vi "RT Loop - System Health and FPGA Monitoring.vi"(10 "FPGA VI Reference":T1, 11 "Message Queue":refnum<queue>) -> ()   [LabVIEW 2018]
uses:
  controls/FPGA VI Reference.ctl
  support/Message Queue/Message Cluster (string).ctl
  controls/FPGA State.ctl
  controls/Raw Values.ctl
  Globals/Global - Configuration Options.vi
  Globals/Global - All RT Loop Stop.vi
  <vilib>/Utility/error.llb/Error Cluster From Error Code.vi
  <vilib>/rvi/errors/niLvFpgaAdjustHostInterfaceError.vi
  <vilib>/nisyscfg/Close (System).vi
  <vilib>/rvi/interface/nirviReadWriteControl/nirviReadWriteControl.xnode
  <vilib>/NI_Real-Time Target Support.lvlib
  <vilib>/nisyscfg/nisyscfg.lvlib
  <resource>/objmgr/nisysapi.rc
  NiFpgaLv.dll
  <vilib>/rvi/interface/Simulation/niFpgaSimulationCallBeginRW.vi
  support/Message Queue/Message Queue.lvlib
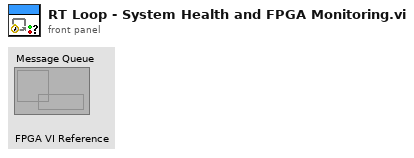
[diagram p1: front panel]
types:
  T1 = typedef "FPGA VI Reference.ctl" = refnum<k20>
  T2 = cluster{"Channel 0":fxp<+/-,20,5>, "Channel 1":fxp<+/-,20,5>, "Channel 2":bool}
  T3 = typedef "NI_Real-Time Target Support.lvlib/RT CPU Load.ctl" = cluster{"Total (%)":dbl, "Time Critical (%)":dbl, "Timed Structures (%)":dbl, "High (%)":dbl, "Above Normal (%)":dbl, "Normal (%)":dbl, "Background (%)":dbl, "Idle (%)":dbl, "ISR (%)":dbl}
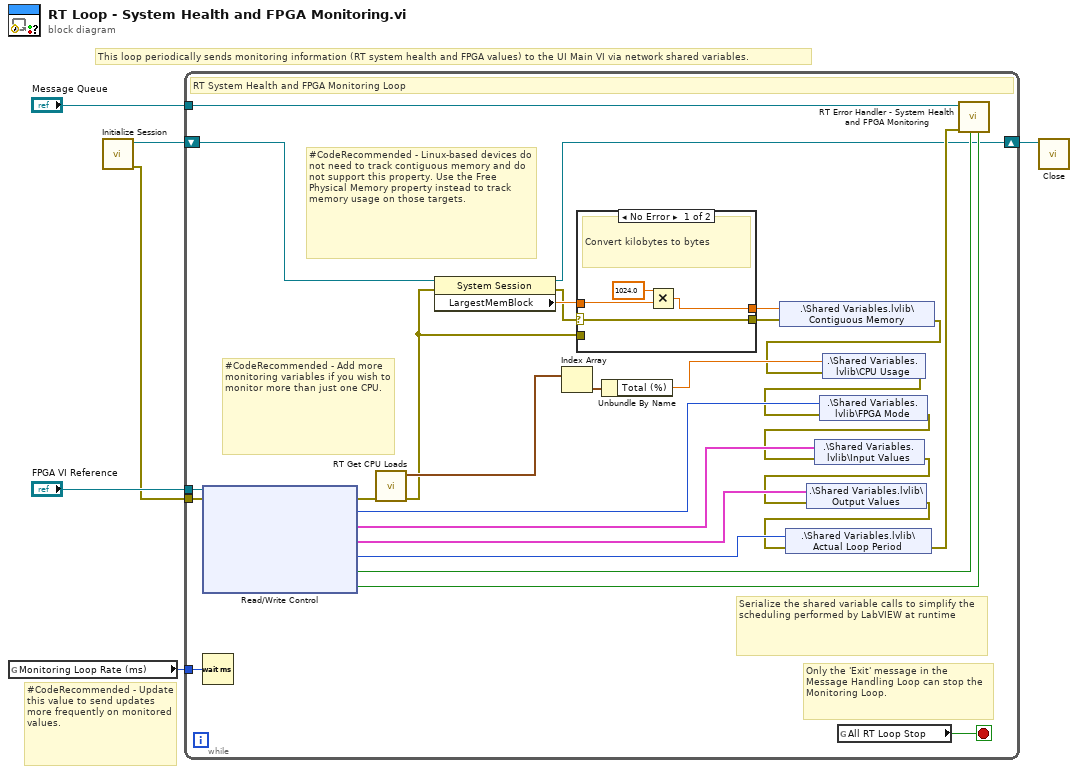
[diagram p0: block diagram]
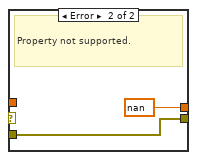
[diagram p2: hidden frame]
diagram:
  # "#CodeRecommended - Update this value to send updates more frequently on monitored values."
  # "This loop periodically sends monitoring information (RT system health and FPGA values) to the UI Main VI via network shared variables."
  n1 = global read "Global - Configuration Options.vi" "Monitoring Loop Rate (ms)"() -> (w4:u32)
  n2 = call <vilib>:"Initialize Session.vi"() -> ("error out"=w1:errorcluster, "Session out"=w3:refnum<k21>)  [unwired: 10 in]
  n3 = while {
    tunnel: "Message Queue" -> [w25]
    tunnel: "FPGA VI Reference" -> [w28]
    tunnel: w4 -> [w24]
    shift-right: [w13] -> w2
    shift-left: w3 -> [w14]
    tunnel: w1 -> [w12]
    stop <- w26 stop-if-true
    # "#CodeRecommended - Linux-based devices do not need to track contiguous memory and do not support this property. Use the Free Physical Memory property instead to track memory usage on those targets."
    # "Serialize the shared variable calls to simplify the scheduling performed by LabVIEW at runtime"
    # "#CodeRecommended - Add more monitoring variables if you wish to monitor more than just one CPU."
    # "Only the 'Exit' message in the  Message Handling Loop can stop the Monitoring Loop."
    # "RT System Health and FPGA Monitoring Loop"
    n4 = xnode "Read/Write Control"("FPGA VI Reference In"=w28, "error in"=w12) -> ("error out"=w21:errorcluster, "Current FPGA State"=w29:enum16{"Safe State", "Control (PID)"}, "Input Values"=w30:T2, "Output Values"=w31:T2, "Actual Loop Period (ticks)"=w27:u32, "Input Error"=w23:bool, "Output Error"=w22:bool)  [unwired: 1 out]
    n5 = Wait (ms)(milliseconds to wait=w24) -> ()  [unwired: 1 out]
    n6 = call <vilib>:"RT Get CPU Loads.vi"("error in (no error)"=w21) -> ("error out"=w8:errorcluster, "CPU loads"=w34:T3[])  [unwired: 9 in]
    n7 = property class="System Session"(reference=w14, error in=w8) -> (reference out=w13:refnum<k21>, error out=w7:errorcluster, "LargestMemBlock"=w9:dbl)
    n8 = Index Array(array=w34) -> (element=w33:T3)  [unwired: 1 in]
    n9 = case shown="No Error" w7 {
      selector: w7 -> [w35 _]
      tunnel: w9 -> [w37 _]
      tunnel: [w36 nan] -> w11
      tunnel: [w35 w39] -> w10
      tunnel: w8 -> [_ w39]
      frame No Error {
        # "Convert kilobytes to bytes"
        n10 = Multiply(x=1024.0, y=w37) -> (x*y=w36:dbl)
      }
      frame Error {
        # "Property not supported."
      }
    }
    n11 = Unbundle By Name(w33) -> ("Total (%)"=w32:dbl)
    n12 = shared-variable ".\\Shared Variables.lvlib\\Contiguous Memory"(w11, error in=w10) -> (error out=w16:errorcluster)
    n13 = shared-variable ".\\Shared Variables.lvlib\\CPU Usage"(w32, error in=w16) -> (error out=w15:errorcluster)
    n14 = shared-variable ".\\Shared Variables.lvlib\\FPGA Mode"(w29, error in=w15) -> (error out=w20:errorcluster)
    n15 = shared-variable ".\\Shared Variables.lvlib\\Input Values"(w30, error in=w20) -> (error out=w19:errorcluster)
    n16 = shared-variable ".\\Shared Variables.lvlib\\Output Values"(w31, error in=w19) -> (error out=w18:errorcluster)
    n17 = shared-variable ".\\Shared Variables.lvlib\\Actual Loop Period"(w27, error in=w18) -> (error out=w17:errorcluster)
    n18 = global read "Global - All RT Loop Stop.vi" "All RT Loop Stop"() -> (w26:bool)
    n19 = call "RT Error Handler - System Health and FPGA Monitoring.vi"("Output Error (FPGA)"=w22, "Input Error (FPGA)"=w23, "error in (no error)"=w17, "Message Queue"=w25) -> ()  [unwired: 7 in, 1 out]
  }
  n20 = call-poly <vilib>:"Close.vi"("Session in"=w2) -> ()  [unwired: 10 in, 1 out]
